vi "Create Action Point.vi"(8 "error in":errorcluster, 9 "Action Point Config from JSON":refnum<class "Config from JSON.lvclass">, 10 "IVritual Instrument":refnum<class "IVirtual Instrument.lvclass">, 11 "ICreate Action Point in":refnum<class "ICreate Action Point.lvclass">) -> (0 "error out":errorcluster, 2 "Action Point out":refnum<class "Action Point.lvclass">, 3 "ICreate Action Point out":refnum<class "ICreate Action Point.lvclass">)   [LabVIEW 2019, in "ICreate Action Point.lvclass"]
uses:
  ICreate Action Point.lvclass
  Action Point/Action Point.lvclass
  Config from JSON/Config from JSON.lvclass
  IVirtual Instrument/IVirtual Instrument.lvclass
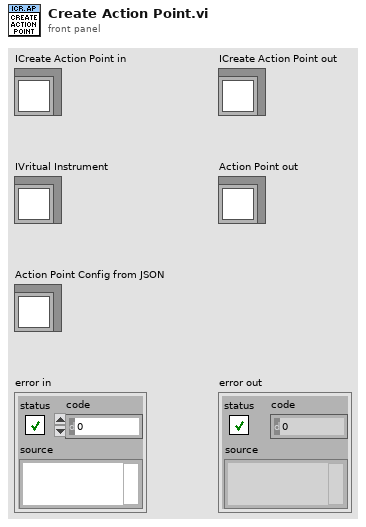
[diagram p1: front panel]
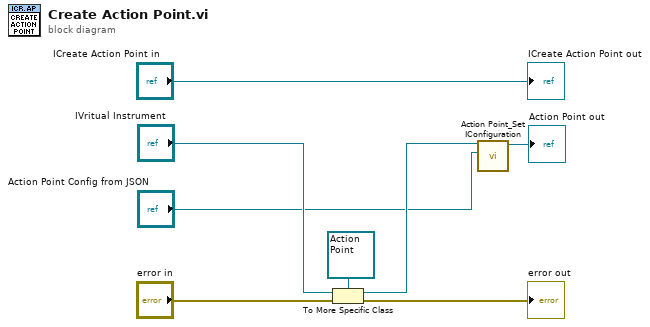
[diagram p0: block diagram]
diagram:
  n1 = To More Specific Class(target class=refnum<class "Action Point.lvclass"> refnum ("specific class reference"), reference="IVritual Instrument", error in="error in") -> (specific class reference=w2:refnum<class "Action Point.lvclass">, error out=→"error out":errorcluster)
  n2 = call "Action Point_Set IConfiguration.vi"("IConfiguration"="Action Point Config from JSON", "Action Point in"=w2) -> ("Action Point out"=→"Action Point out":refnum<class "Action Point.lvclass">)  [unwired: 9 in]
  "ICreate Action Point out" <- "ICreate Action Point in"
